vi "FREQUENCY CONVERSION I.vi"(1 "unit":i32(ring) items=["Hz.", "KHz.", "MHz."], 2 "quantity":ext format="%.2f") -> (0 "output quantity":ext format="%.2f")   [LabVIEW 2025, in "MyDS360.lvlib"]
doc: "This VI is a general purpose VI used to convert the frequency values specified in KHz to the corresponding values in Hz ."
uses:
  MyDS360.lvlib
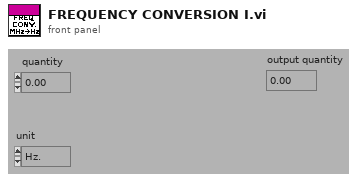
[diagram p1: front panel]
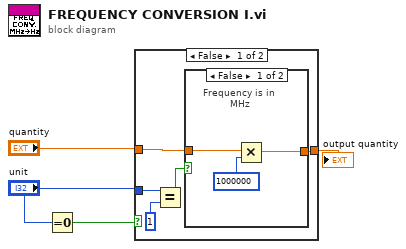
[diagram p0: block diagram]
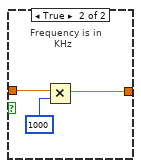
[diagram p2: hidden frame]
diagram:
  n1 = Equal To 0?(x="unit") -> (x = 0?=w2:bool)
  n2 = case shown="False" w2 {
    tunnel: "quantity" -> [w6 w16]
    tunnel: [w5 w16] -> w1
    tunnel: "unit" -> [w9 _]
    frame False {
      n3 = Equal?(x=w9, y=1) -> (x = y?=w7:bool)
      n4 = case shown="False" w7 {
        tunnel: w6 -> [w10 w14]
        tunnel: [w11 w13] -> w5
        frame False {
          # "Frequency is in\n         MHz"
          n5 = Multiply(x=w10, y=1000000) -> (x*y=w11:ext)
        }
        frame True {
          # "Frequency is in\n        KHz"
          n6 = Multiply(x=w14, y=1000) -> (x*y=w13:ext)
        }
      }
    }
    frame True {
      # "Frequency is in Hz"
    }
  }
  "output quantity" <- w1
